vi "AOMindicator.vi"() -> (3 "AOM Ind":cluster{"Photodiode":dbl, "AOM / mV":dbl})   [LabVIEW 2017]
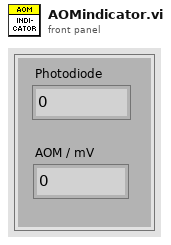
[diagram p1: front panel]
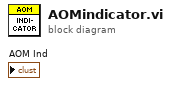
[diagram p0: block diagram]
diagram:
